vi "Error Query.vi"(8 "error in (no error)":errorcluster, 11 "VISA resource name":refnum<visa-resource-name>) -> (0 "error out":errorcluster, 1 "Error Message":string, 2 "Error Code":i32[](array[numeric]), 3 "VISA resource name out":refnum<visa-resource-name>)   [LabVIEW 2021, in "GPT-9000.lvlib"]
doc: "Queries the instrument for any errors in the instrument's error queue. It will continue to read errors until all errors have been read from the instrument. Any errors will be returned in the <B>error out</B> control.\n\n<B>Note:</B>\nThis VI is called automatically by most driver VIs so it is not usually necessary to call this in an application."
uses:
  GPT-9000.lvlib
panel:
  # "EDIT: Note: The Error Query VI is included as a subVI in all driver VIs except low-level API VIs. If the instrument does not support error query, then remove the VI and remove subVI calls in each instrument driver VI that calls it."
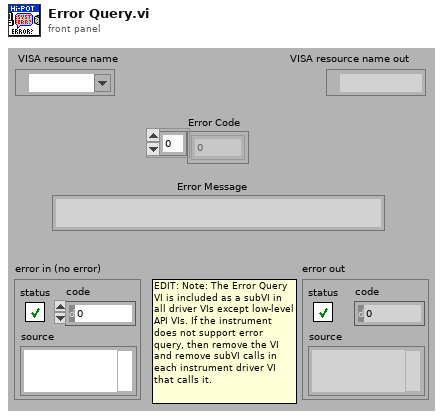
[diagram p1: front panel]
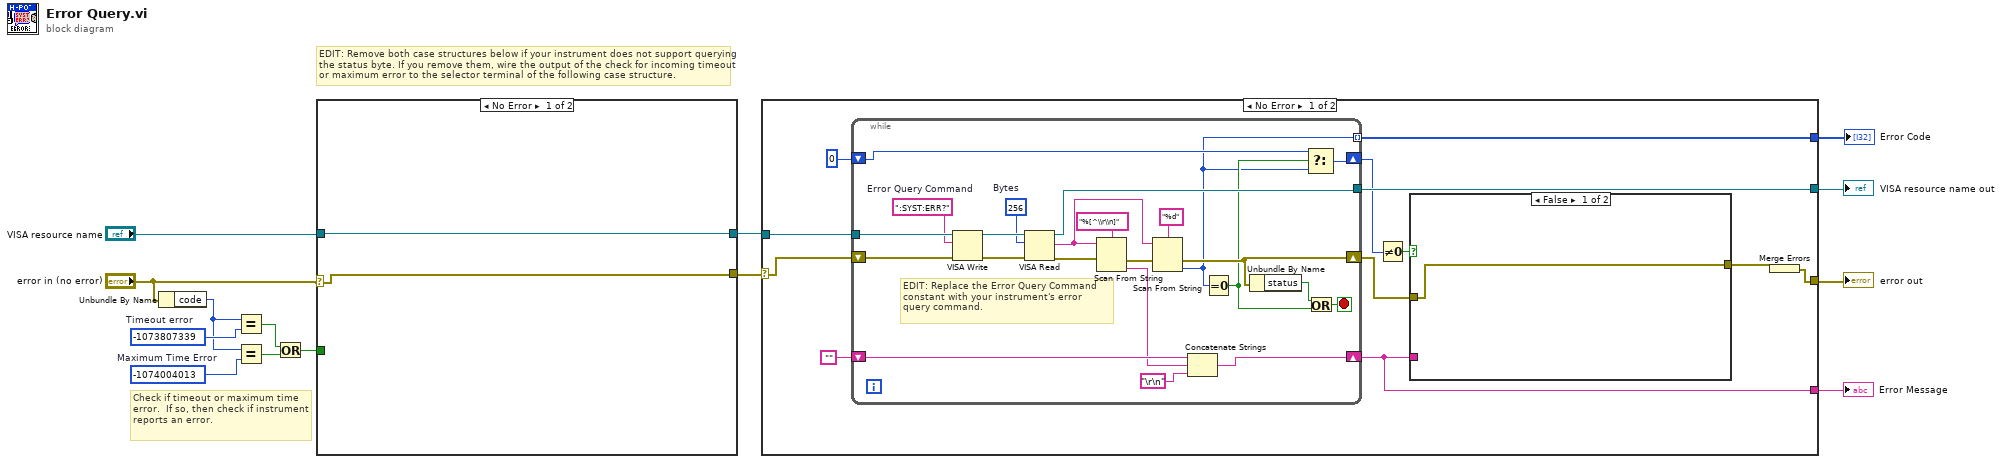
[diagram p0: block diagram]
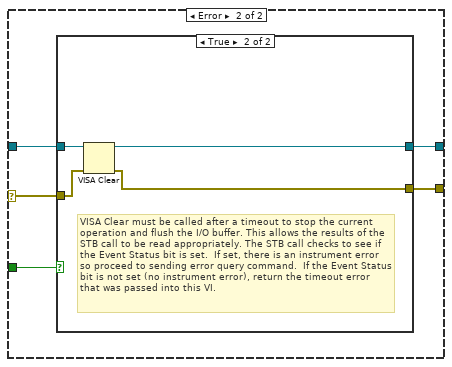
[diagram p2: hidden frame]
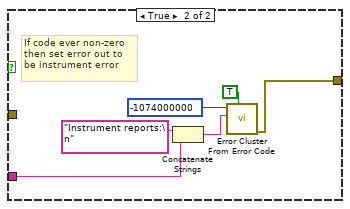
[diagram p4: hidden frame]
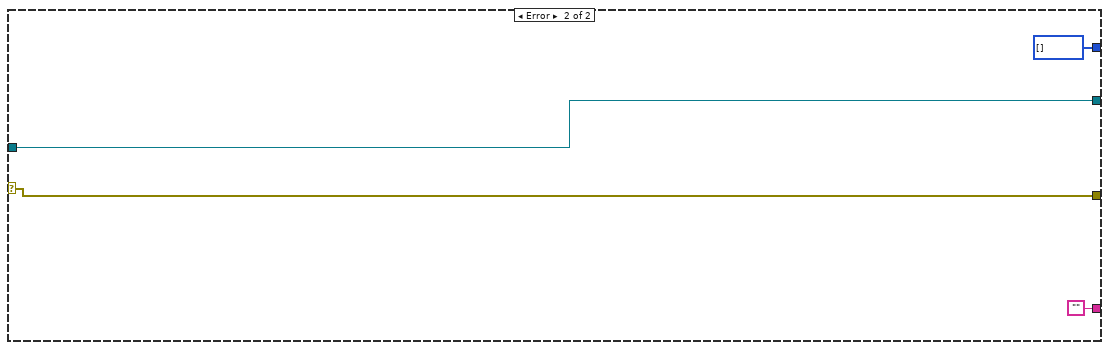
[diagram p5: hidden frame]
diagram:
  w5 = -1074004013  # Maximum Time Error
  w7 = -1073807339  # Timeout error
  # "Check if timeout or maximum time error.  If so, then check if instrument reports an error."
  # "EDIT: Remove both case structures below if your instrument does not support querying the status byte. If you remove them, wire the output of the check for incoming timeout or maximum error to the selector terminal of the following case structure."
  n1 = Unbundle By Name("error in (no error)") -> ("code"=w6:i32)
  n2 = Equal?(x=w6, y=w7) -> (x = y?=w3:bool)
  n3 = Equal?(x=w6, y=w5) -> (x = y?=w4:bool)
  n4 = Or(x=w3, y=w4) -> (x .or. y?=w2:bool)
  n5 = case shown="No Error" "error in (no error)" {
    selector: "error in (no error)" -> [w15 w17]
    tunnel: "VISA resource name" -> [w16 w21]
    tunnel: [w16 w20] -> w9
    tunnel: [w15 w19] -> w10
    tunnel: w2 -> [_ w18]
    frame No Error {
    }
    frame Error {
      n6 = case shown="True" w18 {
        tunnel: w21 -> [w23 w27]
        tunnel: [w23 w26] -> w20
        tunnel: w17 -> [w22 w25]
        tunnel: [w22 w24] -> w19
        frame False {
          # "Error code not a timeout, so best to pass on to user."
        }
        frame True {
          # "VISA Clear must be called after a timeout to stop the current operation and flush the I/O buffer. This allows the results of the  STB call to be read appropriately. The STB call checks to see if the Event Status bit is set.  If set, there is an instrument error so proceed to sending error query command.  If the Event Status bit is not set (no instrument error), return the timeout error that was passed into this VI."
          n7 = VISA Clear(VISA resource name=w27, error in (no error)=w25) -> (VISA resource name out=w26:refnum<visa-resource-name>, error out=w24:errorcluster)
        }
      }
    }
  }
  n8 = case shown="No Error" w10 {
    selector: w10 -> [w28 w70]
    tunnel: [w39 w73] -> w14
    tunnel: w9 -> [w38 w73]
    tunnel: [w36 w70] -> w13
    tunnel: [w31 ""] -> w12
    tunnel: [w30 i32[] []] -> w11
    frame No Error {
      n9 = while {
        tunnel: [w69] -> w39
        tunnel: w38 -> [w68]
        shift-right: [w56] -> w31
        shift-left: "" -> [w59]
        shift-right: [w54] -> w32
        shift-left: 0 -> [w55]
        shift-right: [w52] -> w29
        shift-left: w28 -> [w53]
        tunnel: [w47] -> w30 mode=indexing
        stop <- w62 stop-if-true
        w66 = u32 256  # Bytes
        w64 = ":SYST:ERR?"  # Error Query Command
        # "EDIT: Replace the Error Query Command\nconstant with your instrument's error\nquery command."
        n10 = VISA Write(VISA resource name=w68, write buffer=w64, error in (no error)=w53) -> (VISA resource name out=w67:refnum<visa-resource-name>, error out=w65:errorcluster)  [unwired: 1 out]
        n11 = VISA Read(VISA resource name=w67, byte count=w66, error in (no error)=w65) -> (VISA resource name out=w69:refnum<visa-resource-name>, read buffer=w60:string, error out=w51:errorcluster)  [unwired: 1 out]
        n12 = Scan From String(format string="%[^\\r\\n]", input string=w60, error in=w51) -> (error out=w50:errorcluster, output 1=w57:string)  [unwired: 2 in, 2 out]
        n13 = Scan From String(format string="%d", input string=w60, error in=w50) -> (error out=w52:errorcluster, output 1=w47:i32)  [unwired: 2 in, 2 out]
        n14 = Concatenate Strings(w59, w57, "\r\n") -> (w56:string)
        n15 = Equal To 0?(x=w47) -> (x = 0?=w48:bool)
        n16 = Unbundle By Name(w52) -> ("status"=w49:bool)
        n17 = Select(t=w55, s=w48, f=w47) -> (s? t:f=w54:i32)
        n18 = Or(x=w49, y=w48) -> (x .or. y?=w62:bool)
      }
      n19 = Not Equal To 0?(x=w32) -> (x != 0?=w34:bool)
      n20 = case shown="False" w34 {
        tunnel: w31 -> [_ w45]
        tunnel: [w40 w41] -> w33
        tunnel: w29 -> [w40 _]
        frame False {
        }
        frame True {
          # "If code ever non-zero\nthen set error out to\nbe instrument error"
          n21 = Concatenate Strings("Instrument reports:\n" ("Source"), w45) -> (w42:string)
          n22 = call <vilib>:"Error Cluster From Error Code.vi"("show call chain? (False)"=TRUE, "error message (\"\")"=w42, "error code (0)"=-1074000000 ("Code")) -> ("error out"=w41:errorcluster)  [unwired: 6 in]
        }
      }
      n23 = Merge Errors(w33) -> (w36:errorcluster)
    }
    frame Error {
    }
  }
  "VISA resource name out" <- w14
  "error out" <- w13
  "Error Message" <- w12
  "Error Code" <- w11
